vi "script channels from header.vi"(9 "classifications":T1[](array[typedef]), 10 "types":T2[](array[typedef]), 11 "names":string[](array[string])) -> (3 "channels":refnum<class "TBM channel.lvclass">[](array[class]))   [LabVIEW 2013, in "Shared Library Module configuration.lvclass"]
uses:
  Shared Library Module configuration.lvclass
  <vilib>/NI/Tag Bus/tag/Data Type.ctl
  <vilib>/NI/Tag Bus Module Framework/channel/channel classification.ctl
  <vilib>/NI/Tag Bus Module Framework/channel/TBM channel.lvclass
  <vilib>/NI/Tag Bus/tag/tag descriptor.lvclass
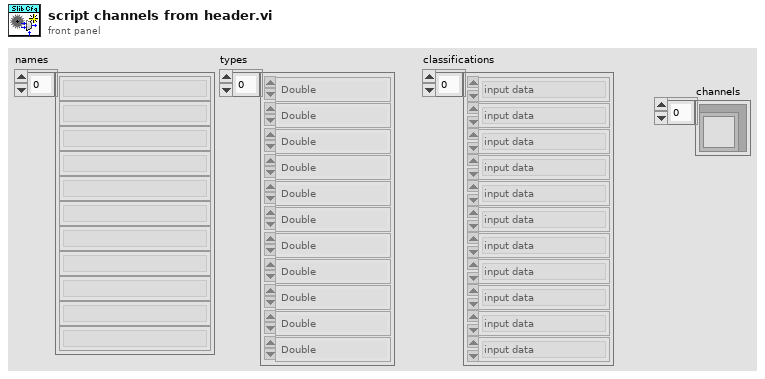
[diagram p1: front panel]
types:
  T1 = typedef "TBM channel.lvclass/channel classification.ctl" = enum16{"input data", "output data", "processing parameter", "processing result"}
  T2 = typedef "tag bus.lvlib/tag descriptor.lvclass/Data Type.ctl" = enum16{"Double", "Single", "I64", "I32", "I16", "I8", "U64", "U32", "U16", "U8", "Boolean", "String", "Array of Double", "Array of Single", "Array of I64", "Array of I32", "Array of I16", "Array of I8", "Array of U64", "Array of U32", "Array of U16", "Array of U8", "Array of Boolean", "Array of String"}
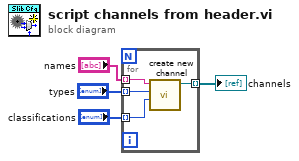
[diagram p0: block diagram]
diagram:
  n1 = for {
    tunnel: "names" -> [w8] mode=indexing
    tunnel: "types" -> [w7] mode=indexing
    tunnel: "classifications" -> [w6] mode=indexing
    tunnel: [w5] -> w1 mode=indexing
    n2 = call <vilib>:"create new channel.vi"("channel classification"=w6, "data type"=w7, "channel name"=w8) -> ("channel"=w5:refnum<class "TBM channel.lvclass">)  [unwired: 8 in]
  }
  "channels" <- w1
